vi "FeedbackDecode_BuildRemotePath.vi"(0 "CompName":string, 1 "FilePattern":string caption="pattern (all files)", 2 "StartPath":path=path "" caption="start path", 5 "DataFolder":string, 7 "TaskName":string, 9 "HeaderName":string caption="pattern (all files)", 11 "ErrorIn":errorcluster) -> (4 "OriginalName":path, 6 "RemoteNetName":path, 8 "RemoteLocalName":path, 10 "FileExt":string, 15 "ErrorOut":errorcluster)   [LabVIEW 2020]
uses:
  <vilib>/regexp/Match Regular Expression.xnode
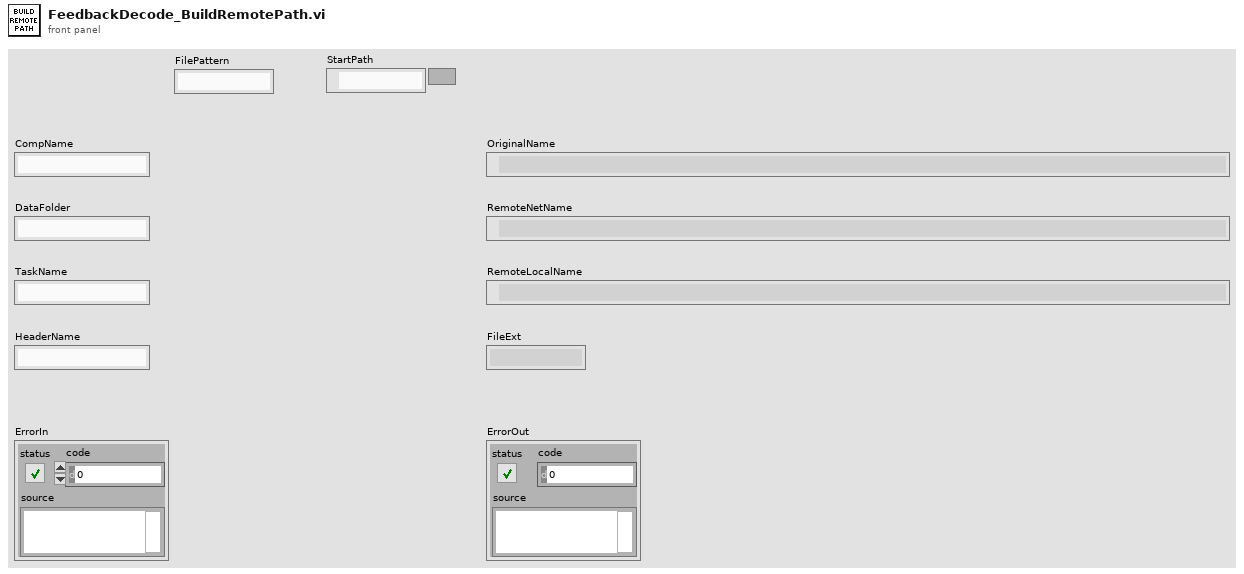
[diagram p1: front panel]
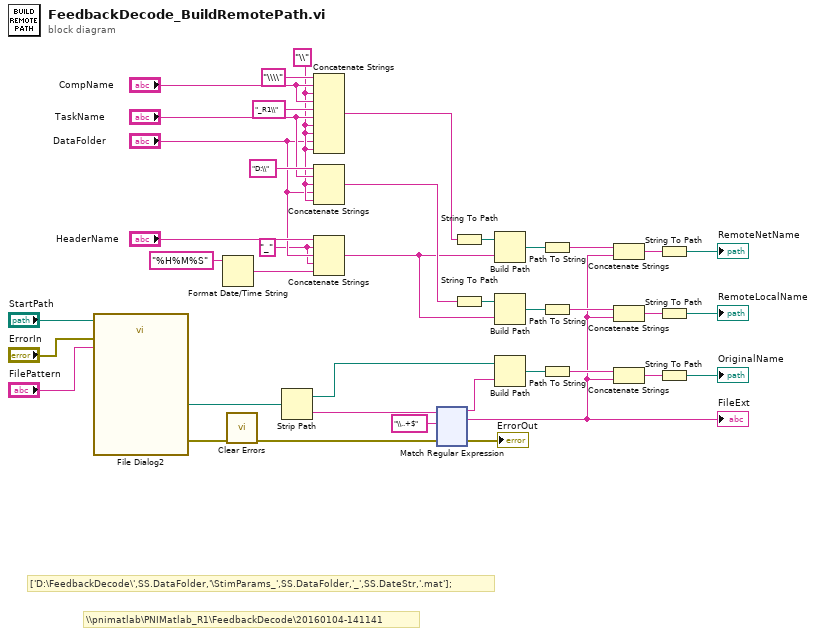
[diagram p0: block diagram]
diagram:
  w28 = "_" ("string")
  w33 = "\\" ("input string")
  # "['D:\\FeedbackDecode\\',SS.DataFolder,'\\StimParams_',SS.DataFolder,'_',SS.DateStr,'.mat'];"
  # "\\\\pnimatlab\\PNIMatlab_R1\\FeedbackDecode\\20160104-141141"
  n1 = call "File Dialog2"("start path"="StartPath", "error in"="ErrorIn", "pattern (all files)"="FilePattern") -> ("selected path"=w23:path, "error out"=w5:errorcluster)  [unwired: 9 in, 2 out]
  n2 = Format Date/Time String(time format string (%c)="%H%M%S") -> (date/time string=w27:string)  [unwired: 2 in]
  n3 = call <vilib>:"Clear Errors.vi"("error in (no error)"=w5) -> ("error out"=w4:errorcluster)  [unwired: 5 in, 1 out]
  n4 = Strip Path(path=w23) -> (stripped path=w19:path, name=w22:string)
  n5 = Concatenate Strings("\\\\" ("input string"), "CompName", w33, "CompName", "_R1\\" ("string"), "TaskName", w33, w33, "DataFolder", w33) -> (w31:string)
  n6 = Concatenate Strings("D:\\" ("string"), "TaskName", w33, "DataFolder", w33) -> (w25:string)
  n7 = Concatenate Strings("HeaderName", w28, "DataFolder", w28, w27) -> (w24:string)
  n8 = xnode "Match Regular Expression"("input string"=w22, "regular expression"="\\..+$", "error in"=w4) -> ("before match"=w20:string, "whole match"=w8:string, "error out"=→"ErrorOut":errorcluster)  [unwired: 3 in, 2 out]
  "FileExt" <- w8
  n9 = String To Path(string=w31) -> (path=w32:path)
  n10 = String To Path(string=w25) -> (path=w26:path)
  n11 = Build Path(base path=w32, name or relative path=w24) -> (appended path=w18:path)
  n12 = Build Path(base path=w26, name or relative path=w24) -> (appended path=w12:path)
  n13 = Build Path(base path=w19, name or relative path=w20) -> (appended path=w10:path)
  n14 = Path To String(path=w18) -> (string=w17:string)
  n15 = Path To String(path=w12) -> (string=w11:string)
  n16 = Path To String(path=w10) -> (string=w9:string)
  n17 = Concatenate Strings(w17, w8) -> (w16:string)
  n18 = Concatenate Strings(w11, w8) -> (w14:string)
  n19 = Concatenate Strings(w9, w8) -> (w13:string)
  n20 = String To Path(string=w16) -> (path=→"RemoteNetName":path)
  n21 = String To Path(string=w14) -> (path=→"RemoteLocalName":path)
  n22 = String To Path(string=w13) -> (path=→"OriginalName":path)
